vi "Excitation Magnitude (Read).vi"(6 "ISOBUS address":T3=-1 caption="ISOBUS address (-1)", 8 "error in":errorcluster, 11 "Mercury Reference In":T4) -> (0 "error out":errorcluster, 1 "Unit":T1, 2 "Excitation Magnitude":dbl, 3 "Mercury Reference Out":T4, 4 "Valid?":T2)   [LabVIEW 2018, in "Mercury iXX.lvlib" / "Temperature.lvlib"]
doc: "Read the current excitation magnitude of the temperature device."
uses:
  Temperature.lvlib
  Mercury Reference.ctl
  Comms Transport Layer.ctl
  Query Dynamic Reference.ctl
  ISOBus Address.ctl
  Is Valid LED.ctl
  Unit String.ctl
  Command Verbs.ctl
  Mercury iXX.lvlib
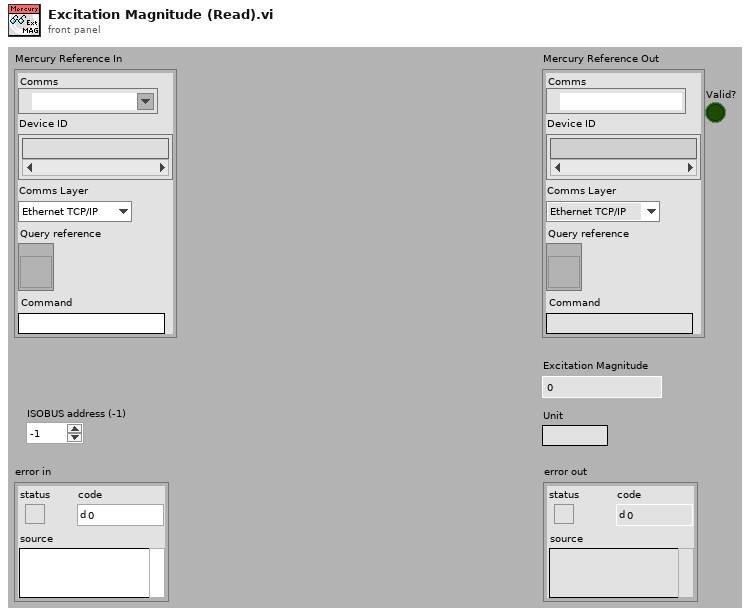
[diagram p1: front panel]
types:
  T1 = typedef "Mercury iXX.lvlib/Unit String.ctl" = string
  T2 = typedef "Mercury iXX.lvlib/Is Valid LED.ctl" = bool
  T3 = typedef "Mercury iXX.lvlib/ISOBus Address.ctl" = i32
  T4 = typedef "Mercury iXX.lvlib/Mercury Reference.ctl" = cluster{"Comms":refnum<visa-resource-name>, "Device ID":string[], "Comms Layer":T5, "Command":string, "Query reference":T6}
  T5 = typedef "Mercury iXX.lvlib/Comms Transport Layer.ctl" = enum16{"Ethernet TCP/IP", "USB", "ISOBus - RS-232", "GPIB"}
  T6 = typedef "Mercury iXX.lvlib/Query Dynamic Reference.ctl" = refnum<vi>
  T7 = typedef "Mercury iXX.lvlib/Command Verbs.ctl" = string
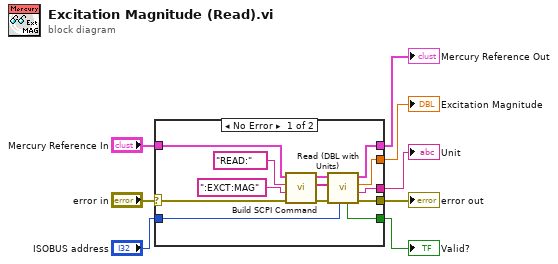
[diagram p0: block diagram]
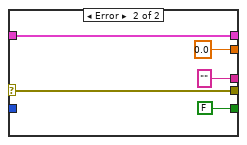
[diagram p2: hidden frame]
diagram:
  n1 = case shown="No Error" "error in" {
    selector: "error in" -> [w11 w26]
    tunnel: "Mercury Reference In" -> [w17 w25]
    tunnel: [w16 w25] -> w7
    tunnel: [w15 w26] -> w6
    tunnel: "ISOBUS address" -> [w14 _]
    tunnel: [w13 T2 FALSE ("Valid?")] -> w4
    tunnel: [w12 0.0 ("Data (Dbl)")] -> w3
    tunnel: [w9 T1 "" ("Unit")] -> w1
    frame No Error {
      n2 = call "Build SCPI Command.vi"("error in"=w11, "Noun(s)"=":EXCT:MAG" ("Command"), "Verb"=T7 "READ:", "Mercury Reference In"=w17) -> ("error out"=w10:errorcluster, "SCPI Message(s)"=w20:string[], "Mercury Reference Out"=w19:T4)  [unwired: 5 out]
      n3 = call "Read (DBL with Units).vi"("ISOBUS address"=w14, "error in"=w10, "SCPI Message(s)"=w20, "Mercury Reference In"=w19) -> ("error out"=w15:errorcluster, "Unit"=w9:T1, "Data (Dbl)"=w12:dbl, "Mercury Reference Out"=w16:T4, "Valid?"=w13:T2)  [unwired: 3 out]
    }
    frame Error {
    }
  }
  "Mercury Reference Out" <- w7
  "error out" <- w6
  "Excitation Magnitude" <- w3
  "Valid?" <- w4
  "Unit" <- w1
